vi "sc5511a_set_reference_dac.vi"(0 "deviceHandle":u32 format="%.0x", 2 "DAC value":u16=57600, 5 "error in":errorcluster) -> (14 "deviceHandle":u32 format="%.0x", 19 "error out":errorcluster)   [LabVIEW 2010]
uses:
  sc5511a.dll
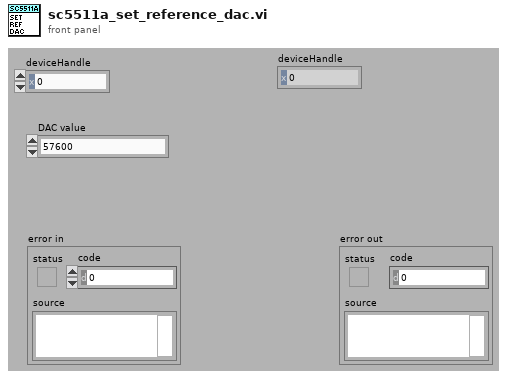
[diagram p1: front panel]
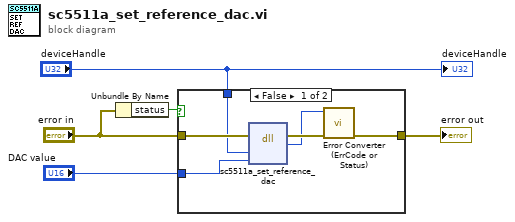
[diagram p0: block diagram]
diagram:
  n1 = Unbundle By Name("error in") -> ("status"=w5:bool)
  n2 = case shown="False" w5 {
    tunnel: "error in" -> [w10 w12]
    tunnel: [w11 w12] -> w3
    tunnel: "deviceHandle" -> [w7 _]
    tunnel: "DAC value" -> [w6 _]
    frame False {
      n3 = dll-call lib="sc5511a.dll" fn="sc5511a_set_reference_dac"(error in=w10, "deviceHandle"=w7, "dac value"=w6) -> (error out=w9:errorcluster, "return type"=w8:i32)  [unwired: 4 in, 1 out]
      n4 = call "Error Converter (ErrCode or Status).vi"("error in (no error)"=w9, "error code"=w8) -> ("error out"=w11:errorcluster)  [unwired: 9 in]
    }
    frame True {
    }
  }
  "error out" <- w3
  "deviceHandle" <- "deviceHandle"
